vi "HFRR ADV v02.vi"() -> ()   [LabVIEW 2025] (continued)
        n1466 = local read "CAMERA ROI MIN TEMP"() -> (w1772:bool)
        n1467 = case shown="True" w1773 {
          selector: w1773 -> [_ w1780]
          frame False {
          }
          frame True {
            n1468 = Not(x=w1780) -> (.not. x?=w1779:bool)
            n1469 = local write "LIVE FEED MIN TEMP"(w1779) -> ()
            n1470 = call "CAMERA LIVE FEED FGV.vi"("Enum - Menu"=CAMERA_LIVE_FEED_ENUM."CAMERA MINIMIZE") -> ()  [unwired: 9 in, 2 out]
          }
        }
        n1471 = case shown="True" w1772 {
          selector: w1772 -> [_ w1777]
          frame False {
          }
          frame True {
            n1472 = Not(x=w1777) -> (.not. x?=w1776:bool)
            n1473 = local write "CAMERA ROI MIN TEMP"(w1776) -> ()
            n1474 = call "IMAGE ANALYSIS.vi"("Enum"=POST_ANALYSIS_ENUM."MINIMIZE UI") -> ()  [unwired: 9 in, 2 out]
          }
        }
        n1475 = local write "CAMERA ROI MAX TEMP"(TRUE ("CAMERA ROI MIN TEMP")) -> ()
      }
      frame "Advance" {
        n1476 = local read "LIVE FEED MIN TEMP"() -> (w1783:bool)
        n1477 = local write "LIVE FEED MAX TEMP"(TRUE ("LIVE FEED MAX TEMP")) -> ()
        n1478 = local read "CAMERA ROI MIN TEMP"() -> (w1781:bool)
        n1479 = case shown="True" w1783 {
          selector: w1783 -> [_ w1790]
          frame False {
          }
          frame True {
            n1480 = Not(x=w1790) -> (.not. x?=w1789:bool)
            n1481 = local write "LIVE FEED MIN TEMP"(w1789) -> ()
            n1482 = call "CAMERA LIVE FEED FGV.vi"("Enum - Menu"=CAMERA_LIVE_FEED_ENUM."CAMERA MINIMIZE") -> ()  [unwired: 9 in, 2 out]
          }
        }
        n1483 = local write "CAMERA ROI MAX TEMP"(TRUE ("CAMERA ROI MAX TEMP")) -> ()
        n1484 = case shown="True" w1781 {
          selector: w1781 -> [_ w1787]
          frame False {
          }
          frame True {
            n1485 = Not(x=w1787) -> (.not. x?=w1786:bool)
            n1486 = local write "CAMERA ROI MIN TEMP"(w1786) -> ()
            n1487 = call "IMAGE ANALYSIS.vi"("Enum"=POST_ANALYSIS_ENUM."MINIMIZE UI") -> ()  [unwired: 9 in, 2 out]
          }
        }
      }
      frame "Mooha" {
        n1488 = local read "LIVE FEED MIN TEMP"() -> (w1793:bool)
        n1489 = local write "LIVE FEED MAX TEMP"(TRUE ("LIVE FEED MAX TEMP")) -> ()
        n1490 = local read "CAMERA ROI MIN TEMP"() -> (w1791:bool)
        n1491 = case shown="True" w1793 {
          selector: w1793 -> [_ w1800]
          frame False {
          }
          frame True {
            n1492 = Not(x=w1800) -> (.not. x?=w1799:bool)
            n1493 = local write "LIVE FEED MIN TEMP"(w1799) -> ()
            n1494 = call "CAMERA LIVE FEED FGV.vi"("Enum - Menu"=CAMERA_LIVE_FEED_ENUM."CAMERA MINIMIZE") -> ()  [unwired: 9 in, 2 out]
          }
        }
        n1495 = local write "CAMERA ROI MAX TEMP"(TRUE ("CAMERA ROI MAX TEMP")) -> ()
        n1496 = case shown="True" w1791 {
          selector: w1791 -> [_ w1797]
          frame False {
          }
          frame True {
            n1497 = Not(x=w1797) -> (.not. x?=w1796:bool)
            n1498 = local write "CAMERA ROI MIN TEMP"(w1796) -> ()
            n1499 = call "IMAGE ANALYSIS.vi"("Enum"=POST_ANALYSIS_ENUM."MINIMIZE UI") -> ()  [unwired: 9 in, 2 out]
          }
        }
      }
    }
    n1500 = local read "Auto Start Test"() -> (w1537:bool)
    n1501 = case shown="True" "sign in temp" {
      frame False {
      }
      frame True {
        w1572 = 1 ("y")
        n1502 = local read "USERNAME"() -> (w1578:string)
        n1503 = local read "USER ID"() -> (w1575:string)
        n1504 = call <vilib>:"Trim Whitespace.vi"("string"=w1578) -> ("trimmed string"=w1577:string)  [unwired: 1 in]
        n1505 = call <vilib>:"Trim Whitespace.vi"("string"=w1575) -> ("trimmed string"=w1576:string)  [unwired: 1 in]
        n1506 = String Length(string=w1577) -> (length=w1574:i32)
        n1507 = String Length(string=w1576) -> (length=w1573:i32)
        n1508 = Greater?(x=w1574, y=w1572) -> (0:w1571:bool)
        n1509 = Greater?(x=w1573, y=w1572) -> (0:w1570:bool)
        n1510 = And(x=w1571, y=w1570) -> (x .and. y?=w1569:bool)
        n1511 = case shown="True" w1569 {
          frame False {
            n1512 = property on="Sign In" class="Bool (strict)"("DisabledEnum"=T19."Disabled" ("Disabled")) -> ()  [unwired: 2 in, 2 out]
          }
          frame True {
            n1513 = property on="Sign In" class="Bool (strict)"("DisabledEnum"=T19."Enabled" ("Disabled")) -> ()  [unwired: 2 in, 2 out]
          }
        }
      }
    }
    n1514 = local read "Air Temperature"() -> (w1554:bool)
    n1515 = local read "Coefficient Of Friction"() -> (w1555:bool)
    n1516 = case shown="False" w1537 {
      frame False {
        n1517 = local read "Auto stop temp"() -> (w1566:bool)
        n1518 = case shown="True" w1566 {
          frame False {
          }
          frame True {
            n1519 = local write "Auto Start Temp"(FALSE ("Auto Start Temp")) -> ()
          }
        }
      }
      frame True {
        "Auto stop temp" <- TRUE ("Auto stop temp")
      }
    }
    n1520 = local read "Humidity 3"() -> (w1553:bool)
    n1521 = case shown="\"HOME\"" w1563 {
      frame "HOME" {
        n1522 = local write "main tab sub"(enum32{"Page 1", "Page 2"}."Page 1" ("main tab sub")) -> ()
      }
      frame Default {
        n1523 = local write "main tab sub"(enum32{"Page 1", "Page 2"}."Page 2" ("main tab sub")) -> ()
      }
    }
    n1524 = case shown="True" w1562 {
      selector: w1562 -> [_ w1915]
      frame False {
      }
      frame True {
        n1525 = Not(x=w1915) -> (.not. x?=w1914:bool)
        n1526 = local write "Sign In"(w1914) -> ()
        n1527 = local write "Main Dashboard Buttons"(T25."Test Setup" ("Main Dashboard Buttons")) -> ()
      }
    }
    n1528 = case shown="\"Graph Display\"" "Num/Graph" {
      frame "Numeric Display", Default {
        n1529 = property on="Single/Multiple" class="RadioBtnsControl (strict)"("Visible"=FALSE) -> ()  [unwired: 2 in, 2 out]
        n1530 = property on="Single - Graph" class="Ring (strict)"("Visible"=FALSE) -> ()  [unwired: 2 in, 2 out]
        n1531 = local write "Main Tab Display"(T6."Dashboard 1" ("Main Tab Display")) -> ()
      }
      frame "Graph Display" {
        n1532 = property on="Single/Multiple" class="RadioBtnsControl (strict)"("Visible"=TRUE) -> ()  [unwired: 2 in, 2 out]
        n1533 = case shown="\"Multiple\"" "Single/Multiple" {
          frame "Single ", Default {
            n1534 = property on="Single - Graph" class="Ring (strict)"("Visible"=TRUE) -> ()  [unwired: 2 in, 2 out]
            n1535 = local write "Main Tab Display"(T6."Dashboard 3" ("Main Tab Display")) -> ()
          }
          frame "Multiple" {
            n1536 = property on="Single - Graph" class="Ring (strict)"("Visible"=FALSE) -> ()  [unwired: 2 in, 2 out]
            n1537 = local write "Main Tab Display"(T6."Dashboard 2" ("Main Tab Display")) -> ()
          }
        }
      }
    }
    n1538 = local read "Stroke"() -> (w1552:bool)
    n1539 = local read "USERNAME"() -> (w1557:string)
    n1540 = case shown="True" w1555 {
      selector: w1555 -> [_ w1840]
      frame False {
      }
      frame True {
        n1541 = Not(x=w1840) -> (.not. x?=w1839:bool)
        n1542 = local write "Coefficient Of Friction"(w1839) -> ()
        n1543 = local write "Tab Control 2"(T8."Coefficient Of Friction" ("Tab Control 2")) -> ()
      }
    }
    n1544 = case shown="True" w1554 {
      selector: w1554 -> [_ w1837]
      frame False {
      }
      frame True {
        n1545 = Not(x=w1837) -> (.not. x?=w1835:bool)
        n1546 = local write "Air Temperature"(w1835) -> ()
        n1547 = local write "Tab Control 2"(T8."Air Temperature" ("Tab Control 2")) -> ()
      }
    }
    n1548 = case shown="True" w1552 {
      selector: w1552 -> [_ w1831]
      frame False {
      }
      frame True {
        n1549 = Not(x=w1831) -> (.not. x?=w1829:bool)
        n1550 = local write "Stroke"(w1829) -> ()
        n1551 = local write "Tab Control 2"(T8."Stroke" ("Tab Control 2")) -> ()
      }
    }
    n1552 = local write "tested by"(w1557) -> ()
    n1553 = case shown="True" w1553 {
      selector: w1553 -> [_ w1834]
      frame False {
      }
      frame True {
        n1554 = Not(x=w1834) -> (.not. x?=w1832:bool)
        n1555 = local write "Humidity 3"(w1832) -> ()
        n1556 = local write "Tab Control 2"(T8."Humidity" ("Tab Control 2")) -> ()
      }
    }
    n1557 = case shown="\"Calibration\"" "Main Dashboard Buttons" {
      tunnel: [T4."HOME" ("Main Tab") T4."Test Setup" ("Main Tab") T4."Acquire" ("Main Tab") T4."Adv Scar" ("Main Tab") T4."Adv Scar Report" ("Main Tab") T4."Compare Files" ("Main Tab") T4."Calibration" ("Main Tab") T4."About" ("Main Tab") T4."Advance" ("Main Tab")] -> w1536
      frame "Home", Default {
      }
      frame "Test Setup" {
      }
      frame "Dashboard" {
      }
      frame "Imaging" {
      }
      frame "Report" {
      }
      frame "Analysis" {
      }
      frame "Calibration" {
      }
      frame "About" {
      }
      frame "Advance" {
      }
    }
    n1558 = Wait (ms)(milliseconds to wait=u32 100) -> ()  [unwired: 1 out]
    n1559 = local read "Main Tab Display"() -> (w1556:T6)
    n1560 = local write "Main Tab"(w1536) -> ()
    n1561 = case shown="\"Dashboard 3\"" w1556 {
      frame "Dashboard 1", Default {
        n1562 = property on="Reset Graph" class="Bool (strict)"("Visible"=FALSE) -> ()  [unwired: 2 in, 2 out]
      }
      frame "Dashboard 2" {
        n1563 = property on="Reset Graph" class="Bool (strict)"("Visible"=TRUE) -> ()  [unwired: 2 in, 2 out]
      }
      frame "Dashboard 3" {
        n1564 = property on="Reset Graph" class="Bool (strict)"("Visible"=TRUE) -> ()  [unwired: 2 in, 2 out]
      }
    }
    n1565 = local read "SCAR MEASURMENT"() -> (w1544:enum32{"Auto Scar", "Manual Scar"})
    n1566 = local read "Humidity"() -> (w1558:bool)
    n1567 = local read "Cap Live Image"() -> (w1541:bool)
    n1568 = local read "Sample Temperature"() -> (w1551:bool)
    n1569 = local read "Air Temp vs Humidity"() -> (w1549:bool)
    n1570 = local read "Frequency"() -> (w1550:bool)
    n1571 = case shown="False" w1558 {
      frame False {
        n1572 = local write "Humidity On Command"(TRUE ("Humidity On Command")) -> ()
        n1573 = case shown="True" "Humidity Off Command" {
          selector: "Humidity Off Command" -> [_ w1847]
          frame False {
          }
          frame True {
            n1574 = stacked-sequence {
              frame #0 {
                n1575 = local read "WriteHumidity"() -> (w1849:string[])
                n1576 = Insert Into Array(array=w1849, new element="R;1" ("new element/subarray")) -> (w1848:string[])  [unwired: 1 in]
                n1577 = local write "WriteHumidity"(w1848) -> ()
              }
              frame #1 {
                n1578 = Wait (ms)(milliseconds to wait=u32 500) -> ()  [unwired: 1 out]
              }
              frame #2 {
                n1579 = local read "WriteHumidity"() -> (w1853:string[])
                n1580 = local read "EVENT LOG"() -> (w1857:string)
                n1581 = call "Event Log.vi"("Content"="Humidity Control Off" ("string"), "EVENT LOG"=w1857) -> ("EVENT LOG"=w1858:string)  [unwired: 8 in, 1 out]
                n1582 = local write "EVENT LOG"(w1858) -> ()
                n1583 = Insert Into Array(array=w1853, new element="R;1" ("new element/subarray")) -> (w1854:string[])  [unwired: 1 in]
                n1584 = local write "WriteHumidity"(w1854) -> ()
                n1585 = local write "Humidity 2"(TRUE ("Humidity")) -> ()
              }
            }
            n1586 = Not(x=w1847) -> (.not. x?=w1846:bool)
            n1587 = local write "Humidity Off Command"(w1846) -> ()
          }
        }
      }
      frame True {
        n1588 = local write "Humidity Off Command"(TRUE ("Humidity Off Command")) -> ()
        n1589 = case shown="False" "Humidity On Command" {
          selector: "Humidity On Command" -> [_ w1862]
          frame False {
          }
          frame True {
            n1590 = stacked-sequence {
              frame #0 {
                n1591 = local read "Set Rh"() -> (w1868:dbl)
                n1592 = local read "WriteHumidity"() -> (w1864:string[])
                n1593 = Number To Fractional String(number=w1868, precision (6)=i16 2) -> (F-format string=w1869:string)  [unwired: 2 in]
                n1594 = Concatenate Strings("M;" ("new element/subarray"), w1869) -> (w1867:string)
                n1595 = Insert Into Array(array=w1864, new element=w1867) -> (w1863:string[])  [unwired: 1 in]
                n1596 = local write "WriteHumidity"(w1863) -> ()
              }
              frame #1 {
                n1597 = Wait (ms)(milliseconds to wait=u32 500) -> ()  [unwired: 1 out]
              }
              frame #2 {
                n1598 = local read "WriteHumidity"() -> (w1872:string[])
                n1599 = local read "Set Rh"() -> (w1876:dbl)
                n1600 = Number To Fractional String(number=w1876, precision (6)=i16 2) -> (F-format string=w1877:string)  [unwired: 2 in]
                n1601 = Concatenate Strings("M;" ("new element/subarray"), w1877) -> (w1875:string)
                n1602 = Insert Into Array(array=w1872, new element=w1875) -> (w1871:string[])  [unwired: 1 in]
                n1603 = local write "WriteHumidity"(w1871) -> ()
              }
              frame #3 {
                n1604 = Wait (ms)(milliseconds to wait=u32 500) -> ()  [unwired: 1 out]
              }
              frame #4 {
                (unwired) "% RH" ("string")
                (unwired) i16 2 ("precision (6)")
                (unwired) "M;" ("new element/subarray")
                n1605 = local read "Set Rh"() -> (w1886:dbl)
                n1606 = local read "WriteHumidity"() -> (w1879:string[])
                n1607 = Number To Fractional String(number=w1886, precision (6)=i16 2) -> (F-format string=w1883:string)  [unwired: 2 in]
                n1608 = Concatenate Strings("M;" ("new element/subarray"), w1883) -> (w1887:string)
                n1609 = Concatenate Strings("Humidity Set to : " ("string"), w1883, "% RH" ("string")) -> (w1881:string)
                n1610 = Insert Into Array(array=w1879, new element=w1887) -> (w1880:string[])  [unwired: 1 in]
                n1611 = disable-structure shown="Enabled" {
                  frame Enabled {
                    n1612 = local read "EVENT LOG"() -> (w1890:string)
                    n1613 = call "Event Log.vi"("Content"="Humidity Control On", "EVENT LOG"=w1890) -> ("EVENT LOG"=w1891:string)  [unwired: 8 in, 1 out]
                    n1614 = local write "EVENT LOG"(w1891) -> ()
                  }
                  frame Disabled {
                  }
                }
                n1615 = disable-structure shown="Enabled" {
                  disable-tunnel: w1881 -> [_ _]
                  frame Enabled {
                    n1616 = local read "EVENT LOG"() -> (w1893:string)
                    n1617 = call "Event Log.vi"("Content"="Humidity Control On", "EVENT LOG"=w1893) -> ("EVENT LOG"=w1894:string)  [unwired: 8 in, 1 out]
                    n1618 = local write "EVENT LOG"(w1894) -> ()
                  }
                  frame Disabled {
                  }
                }
                n1619 = local write "WriteHumidity"(w1880) -> ()
              }
            }
            n1620 = Not(x=w1862) -> (.not. x?=w1861:bool)
            n1621 = local write "Humidity On Command"(w1861) -> ()
          }
        }
      }
    }
    n1622 = Equal?(x=w1544, y=enum32{"Auto Scar", "Manual Scar"}."Auto Scar" ("SCAR MEASURMENT")) -> (x = y?=w1540:bool)
    n1623 = local read "TEST STANDARD"() -> (w1547:T5)
    n1624 = And(x=w1541, y=w1540) -> (x .and. y?=w1542:bool)
    n1625 = case shown="True" w1542 {
      selector: w1542 -> [_ w1645]
      tunnel: errorcluster {"status"=FALSE, "code"=0, "source"=""} ("error in (no error) 3") -> [_ w1646]
      frame False {
      }
      frame True {
        n1626 = stacked-sequence {
          tunnel: w1646 -> [_ _ _ _ _ _ _ w1695]
          tunnel: w1645 -> [_ _ _ _ _ w1675 _ _]
          frame #0 {
            n1627 = call "CAMERA LIVE FEED FGV.vi"("Enum - Menu"=CAMERA_LIVE_FEED_ENUM."CAMERA MINIMIZE") -> ()  [unwired: 9 in, 2 out]
          }
          frame #1 {
            n1628 = property on="Auto Scar Check  2" class="Clust (strict)"("Visible"=TRUE) -> ()  [unwired: 2 in, 2 out]
          }
          frame #2 {
            n1629 = String To Path(string="C:\\LAB-IQ\\Image Calibrate v01.dcf") -> (path=w1651:path)
            n1630 = Open/Create/Replace File ("Open File")(file path (use dialog)=w1651) -> (refnum out=w1652:refnum<file>)  [unwired: 5 in, 2 out]
            n1631 = for {
              N: 4 -> [_]
              tunnel: w1652 -> [w1658]
              i -> [w1654]
              n1632 = Read from Text File ("Read File")(file (use dialog)=w1658) -> (text=w1659:string)  [unwired: 3 in, 3 out]
              n1633 = String Subset(string=w1659, offset (0)=6, length (rest)=10 ("length (rest)")) -> (substring=w1655:string)
              n1634 = Fract/Exp String To Number(string=w1655) -> (number=w1653:dbl)  [unwired: 3 in, 1 out]
              n1635 = case shown="0" w1654 {
                tunnel: w1653 -> [w1660 w1661 _ w1662 _]
                frame 0 {
                  "5x Gain" <- w1660
                }
                frame 1 {
                  "10x Gain" <- w1661
                }
                frame 2 {
                }
                frame 3 {
                  "100x gain" <- w1662
                }
                frame 4, Default {
                }
              }
            }
          }
          frame #3 {
            n1636 = local read "FILE 3"() -> (w1668:string)
            n1637 = call <vilib>:"Trim Whitespace.vi"("string"="C:\\LAB-IQ\\images\\") -> ("trimmed string"=w1670:string)  [unwired: 1 in]
            n1638 = String To Path(string=w1670) -> (path=w1669:path)
            n1639 = Concatenate Strings(w1668, ".png" ("string")) -> (w1667:string)
            n1640 = Build Path(base path=w1669, name or relative path=w1667) -> (appended path=w1665:path)
            "Image path" <- w1665
            n1641 = Path To String(path=w1665) -> (string=w1664:string)
            n1642 = call "CAMERA LIVE FEED FGV.vi"("Enum - Menu"=CAMERA_LIVE_FEED_ENUM."CAMERA SAVE", "Image Path"=w1664) -> ()  [unwired: 8 in, 2 out]
          }
          frame #4 {
            n1643 = One Button Dialog(message="Image saved successfully") -> ()  [unwired: 1 in, 1 out]
          }
          frame #5 {
            n1644 = local read "TEST STANDARD"() -> (w1674:T5)
            n1645 = local read "Magnification len live scar"() -> (w1686:string)
            n1646 = Not(x=w1675) -> (.not. x?=w1676:bool)
            n1647 = local write "Cap Live Image"(w1676) -> ()
            n1648 = case shown="\"ASTM D7688\"" w1674 {
              tunnel: ["ASTM D6079" "ISO 12156" "ASTM D7688"] -> w1673
              frame "ASTM D6079", Default {
              }
              frame "ISO 12156" {
              }
              frame "ASTM D7688" {
              }
            }
            n1649 = case shown="\"5x\", Default" w1686 {
              tunnel: [w1690 w1691] -> w1685
              frame "5x", Default {
                n1650 = local read "5x Gain"() -> (w1690:dbl)
              }
              frame "10x" {
                # "5x"
                n1651 = local read "10x Gain"() -> (w1691:dbl)
              }
            }
            n1652 = local read "Image path"() -> (w1684:path)
            n1653 = local read "FILE 3"() -> (w1677:string)
            n1654 = call "EDGE DETCTION.vi"("GAIN VALUE"=w1685, "Image Path"=w1684) -> ("error out"=w1683:errorcluster, "return value"=w1682:cluster{string, string, dbl, dbl, dbl})  [unwired: 8 in]
            n1655 = Bundle By Name(cluster=T26 {"File Name"="", "Test Method"="", "Operator"="", "Fuel Description"="", "Date and time"=""} ("Main Ref"), "File Name"=w1677, "Test Method"=w1673) -> (w1678:T26)
            n1656 = call "duf file read.vi"("error in (no error)"=w1683, "Main Ref"=w1678) -> ("error out"=w1681:errorcluster, "Main Ref 2"=w1679:T26)  [unwired: 7 in, 1 out]
            n1657 = call "EDGE DETECTION REPORT.vi"("error in (no error)"=w1681, "return value 2"=w1682, "Main Ref"=w1679) -> ()  [unwired: 8 in, 1 out]
          }
          frame #6 {
            n1658 = property on="Auto Scar Check  2" class="Clust (strict)"("Visible"=FALSE) -> ()  [unwired: 2 in, 2 out]
          }
          frame #7 {
            n1659 = call "CAMERA LIVE FEED FGV.vi"("Enum - Menu"=CAMERA_LIVE_FEED_ENUM."CAMERA MINIMIZE", "error in (no error)"=w1695) -> ()  [unwired: 8 in, 2 out]
            n1660 = local write "Main Dashboard Buttons"(T1."Home" ("Main Dashboard Buttons")) -> ()
            n1661 = local write "Main Tab"(T4."HOME" ("Main Tab")) -> ()
          }
        }
      }
    }
    n1662 = local read "Heater Button"() -> (w1548:bool)
    n1663 = case shown="True" w1550 {
      selector: w1550 -> [_ w1825]
      frame False {
      }
      frame True {
        n1664 = Not(x=w1825) -> (.not. x?=w1823:bool)
        n1665 = local write "Frequency"(w1823) -> ()
        n1666 = local write "Tab Control 2"(T8."Frequency" ("Tab Control 2")) -> ()
      }
    }
    n1667 = case shown="True" w1549 {
      selector: w1549 -> [_ w1822]
      frame False {
      }
      frame True {
        n1668 = Not(x=w1822) -> (.not. x?=w1820:bool)
        n1669 = local write "Air Temp vs Humidity"(w1820) -> ()
        n1670 = local write "Tab Control 2"(T8."Air Temp vs Rh" ("Tab Control 2")) -> ()
      }
    }
    n1671 = case shown="True" w1551 {
      selector: w1551 -> [_ w1828]
      frame False {
      }
      frame True {
        n1672 = Not(x=w1828) -> (.not. x?=w1826:bool)
        n1673 = local write "Sample Temperature"(w1826) -> ()
        n1674 = local write "Tab Control 2"(T8."Sample Temperature" ("Tab Control 2")) -> ()
      }
    }
    n1675 = case shown="\"ASTM D7688\"" w1547 {
      frame "ASTM D6079", Default {
        w1801 = "ASTM D6079 TEST CONDITIONS" ("Standard 2")
        n1676 = local write "Standard 2"(w1801) -> ()
        n1677 = local write "Standard"(w1801) -> ()
      }
      frame "ISO 12156" {
        w1802 = "ISO 12156 TEST CONDITIONS" ("Standard 2")
        n1678 = local write "Standard 2"(w1802) -> ()
        n1679 = local write "Standard"(w1802) -> ()
      }
      frame "ASTM D7688" {
        w1803 = "ASTM D7688 TEST CONDITIONS" ("Standard 2")
        n1680 = local write "Standard 2"(w1803) -> ()
        n1681 = local write "Standard"(w1803) -> ()
      }
      frame "Custom" {
        w1804 = "CUSTOM TEST CONDITIONS" ("Standard 2")
        n1682 = local write "Standard 2"(w1804) -> ()
        n1683 = local write "Standard"(w1804) -> ()
      }
    }
    n1684 = case shown="True" w1548 {
      frame False {
        n1685 = local write "Temperature On Command"(TRUE ("Temperature On Command")) -> ()
        n1686 = case shown="True" "Temperature Off Command" {
          selector: "Temperature Off Command" -> [_ w1808]
          frame False {
          }
          frame True {
            n1687 = Not(x=w1808) -> (.not. x?=w1807:bool)
            n1688 = local read "EVENT LOG"() -> (w1811:string)
            n1689 = local write "Temperature Off Command"(w1807) -> ()
            n1690 = call "Event Log.vi"("Content"="Heater Off", "EVENT LOG"=w1811) -> ("EVENT LOG"=w1810:string)  [unwired: 8 in, 1 out]
            n1691 = local write "EVENT LOG"(w1810) -> ()
          }
        }
      }
      frame True {
        n1692 = local write "Temperature Off Command"(TRUE ("Temperature Off Command")) -> ()
        n1693 = case shown="True" "Temperature On Command" {
          selector: "Temperature On Command" -> [_ w1815]
          frame False {
          }
          frame True {
            n1694 = Not(x=w1815) -> (.not. x?=w1814:bool)
            n1695 = local write "Temperature On Command"(w1814) -> ()
            n1696 = disable-structure shown="Enabled" {
              disable-tunnel: "Heater On" -> [w1817 _]
              frame Enabled {
                n1697 = local read "EVENT LOG"() -> (w1818:string)
                n1698 = call "Event Log.vi"("Content"=w1817, "EVENT LOG"=w1818) -> ("EVENT LOG"=w1819:string)  [unwired: 8 in, 1 out]
                n1699 = local write "EVENT LOG"(w1819) -> ()
              }
              frame Disabled {
              }
            }
          }
        }
      }
    }
    n1700 = local read "Main Tab"() -> (w1539:T4)
    n1701 = case shown="\"About\"" w1539 {
      frame "HOME", Default {
        w1581 = T19."Enabled" ("Disabled")
        n1702 = local read "Service Password enable"() -> (w1583:bool)
        n1703 = property on="Imaging" class="Bool (strict)"("DisabledEnum"=w1581) -> ()  [unwired: 2 in, 2 out]
        n1704 = property on="Dashboard" class="Bool (strict)"("DisabledEnum"=w1581) -> ()  [unwired: 2 in, 2 out]
        n1705 = property on="Test Setup" class="Bool (strict)"("DisabledEnum"=w1581) -> ()  [unwired: 2 in, 2 out]
        n1706 = property on="Analysis" class="Bool (strict)"("DisabledEnum"=w1581) -> ()  [unwired: 2 in, 2 out]
        n1707 = property on="Home" class="Bool (strict)"("DisabledEnum"=w1581) -> ()  [unwired: 2 in, 2 out]
        n1708 = property on="Report" class="Bool (strict)"("DisabledEnum"=w1581) -> ()  [unwired: 2 in, 2 out]
        n1709 = property on="Main Dashboard Buttons" class="RadioBtnsControl (strict)"("DisabledEnum"=w1581) -> ()  [unwired: 2 in, 2 out]
        n1710 = property on="Calibration" class="Bool (strict)"("DisabledEnum"=w1581) -> ()  [unwired: 2 in, 2 out]
        n1711 = case shown="True" w1583 {
          tunnel: [T19."Disabled" ("Disabled") T19."Enabled" ("Disabled")] -> w1582
          frame False {
          }
          frame True {
          }
        }
        n1712 = property on="About" class="Bool (strict)"("DisabledEnum"=w1582) -> ()  [unwired: 2 in, 2 out]
      }
      frame "Test Setup" {
        w1588 = T19."Enabled" ("Disabled")
        n1713 = local read "Service Password enable"() -> (w1587:bool)
        n1714 = property on="Dashboard" class="Bool (strict)"("DisabledEnum"=T19."Disabled" ("Disabled")) -> ()  [unwired: 2 in, 2 out]
        n1715 = property on="Imaging" class="Bool (strict)"("DisabledEnum"=w1588) -> ()  [unwired: 2 in, 2 out]
        n1716 = property on="Analysis" class="Bool (strict)"("DisabledEnum"=w1588) -> ()  [unwired: 2 in, 2 out]
        n1717 = property on="Home" class="Bool (strict)"("DisabledEnum"=w1588) -> ()  [unwired: 2 in, 2 out]
        n1718 = property on="Report" class="Bool (strict)"("DisabledEnum"=w1588) -> ()  [unwired: 2 in, 2 out]
        n1719 = property on="Test Setup" class="Bool (strict)"("DisabledEnum"=w1588) -> ()  [unwired: 2 in, 2 out]
        n1720 = case shown="True" w1587 {
          tunnel: [T19."Disabled" ("Disabled") T19."Enabled" ("Disabled")] -> w1586
          frame False {
          }
          frame True {
          }
        }
        n1721 = property on="About" class="Bool (strict)"("DisabledEnum"=w1586) -> ()  [unwired: 2 in, 2 out]
      }
      frame "Adv Scar" {
        w1595 = T19."Enabled" ("Disabled")
        n1722 = property on="Dashboard" class="Bool (strict)"("DisabledEnum"=T19."Disabled" ("Disabled")) -> ()  [unwired: 2 in, 2 out]
        n1723 = property on="Imaging" class="Bool (strict)"("DisabledEnum"=w1595) -> ()  [unwired: 2 in, 2 out]
        n1724 = property on="Analysis" class="Bool (strict)"("DisabledEnum"=w1595) -> ()  [unwired: 2 in, 2 out]
        n1725 = property on="Home" class="Bool (strict)"("DisabledEnum"=w1595) -> ()  [unwired: 2 in, 2 out]
        n1726 = property on="Report" class="Bool (strict)"("DisabledEnum"=w1595) -> ()  [unwired: 2 in, 2 out]
        n1727 = property on="Test Setup" class="Bool (strict)"("DisabledEnum"=w1595) -> ()  [unwired: 2 in, 2 out]
        n1728 = local read "Service Password enable"() -> (w1593:bool)
        n1729 = case shown="True" w1593 {
          tunnel: [T19."Disabled" ("Disabled") T19."Enabled" ("Disabled")] -> w1592
          frame False {
          }
          frame True {
          }
        }
        n1730 = property on="About" class="Bool (strict)"("DisabledEnum"=w1592) -> ()  [unwired: 2 in, 2 out]
      }
      frame "Calibration" {
        w1598 = T19."Enabled" ("Disabled")
        n1731 = property on="Dashboard" class="Bool (strict)"("DisabledEnum"=T19."Disabled" ("Disabled")) -> ()  [unwired: 2 in, 2 out]
        n1732 = property on="Imaging" class="Bool (strict)"("DisabledEnum"=w1598) -> ()  [unwired: 2 in, 2 out]
        n1733 = property on="Analysis" class="Bool (strict)"("DisabledEnum"=w1598) -> ()  [unwired: 2 in, 2 out]
        n1734 = property on="Home" class="Bool (strict)"("DisabledEnum"=w1598) -> ()  [unwired: 2 in, 2 out]
        n1735 = property on="Report" class="Bool (strict)"("DisabledEnum"=w1598) -> ()  [unwired: 2 in, 2 out]
        n1736 = property on="Test Setup" class="Bool (strict)"("DisabledEnum"=w1598) -> ()  [unwired: 2 in, 2 out]
        n1737 = local read "Service Password enable"() -> (w1600:bool)
        n1738 = property on="Calibration" class="Bool (strict)"("DisabledEnum"=w1598) -> ()  [unwired: 2 in, 2 out]
        n1739 = case shown="True" w1600 {
          tunnel: [T19."Disabled" ("Disabled") T19."Enabled" ("Disabled")] -> w1599
          frame False {
          }
          frame True {
          }
        }
        n1740 = property on="About" class="Bool (strict)"("DisabledEnum"=w1599) -> ()  [unwired: 2 in, 2 out]
      }
      frame "Adv Scar Report" {
        w1606 = T19."Enabled" ("Disabled")
        n1741 = property on="Dashboard" class="Bool (strict)"("DisabledEnum"=T19."Disabled" ("Disabled")) -> ()  [unwired: 2 in, 2 out]
        n1742 = property on="Imaging" class="Bool (strict)"("DisabledEnum"=w1606) -> ()  [unwired: 2 in, 2 out]
        n1743 = property on="Analysis" class="Bool (strict)"("DisabledEnum"=w1606) -> ()  [unwired: 2 in, 2 out]
        n1744 = property on="Home" class="Bool (strict)"("DisabledEnum"=w1606) -> ()  [unwired: 2 in, 2 out]
        n1745 = property on="Report" class="Bool (strict)"("DisabledEnum"=w1606) -> ()  [unwired: 2 in, 2 out]
        n1746 = property on="Test Setup" class="Bool (strict)"("DisabledEnum"=w1606) -> ()  [unwired: 2 in, 2 out]
        n1747 = local read "Service Password enable"() -> (w1605:bool)
        n1748 = case shown="True" w1605 {
          tunnel: [T19."Disabled" ("Disabled") T19."Enabled" ("Disabled")] -> w1604
          frame False {
          }
          frame True {
          }
        }
        n1749 = property on="About" class="Bool (strict)"("DisabledEnum"=w1604) -> ()  [unwired: 2 in, 2 out]
      }
      frame "Compare Files" {
        w1612 = T19."Enabled" ("Disabled")
        n1750 = local read "Service Password enable"() -> (w1611:bool)
        n1751 = property on="Dashboard" class="Bool (strict)"("DisabledEnum"=T19."Disabled" ("Disabled")) -> ()  [unwired: 2 in, 2 out]
        n1752 = property on="Imaging" class="Bool (strict)"("DisabledEnum"=w1612) -> ()  [unwired: 2 in, 2 out]
        n1753 = property on="Analysis" class="Bool (strict)"("DisabledEnum"=w1612) -> ()  [unwired: 2 in, 2 out]
        n1754 = property on="Home" class="Bool (strict)"("DisabledEnum"=w1612) -> ()  [unwired: 2 in, 2 out]
        n1755 = property on="Report" class="Bool (strict)"("DisabledEnum"=w1612) -> ()  [unwired: 2 in, 2 out]
        n1756 = property on="Test Setup" class="Bool (strict)"("DisabledEnum"=w1612) -> ()  [unwired: 2 in, 2 out]
        n1757 = case shown="True" w1611 {
          tunnel: [T19."Disabled" ("Disabled") T19."Enabled" ("Disabled")] -> w1610
          frame False {
          }
          frame True {
          }
        }
        n1758 = property on="About" class="Bool (strict)"("DisabledEnum"=w1610) -> ()  [unwired: 2 in, 2 out]
      }
      frame "Acquire" {
        n1759 = local read "Service Password enable"() -> (w1617:bool)
        n1760 = property on="Test Setup" class="Bool (strict)"("DisabledEnum"=T19."Disabled" ("Disabled")) -> ()  [unwired: 2 in, 2 out]
        n1761 = local read "Auto Start Test"() -> (w1619:bool)
        n1762 = local read "RUN"() -> (w1621:bool)
        n1763 = case shown="True" w1617 {
          tunnel: [T19."Disabled" ("Disabled") T19."Enabled" ("Disabled")] -> w1618
          frame False {
          }
          frame True {
          }
        }
        n1764 = Or(x=w1621, y=w1619) -> (x .or. y?=w1620:bool)
        n1765 = case shown="True" w1620 {
          tunnel: [T19."Enabled" ("Disabled") T19."Disabled" ("Disabled")] -> w1616
          frame False {
          }
          frame True {
          }
        }
        n1766 = property on="About" class="Bool (strict)"("DisabledEnum"=w1618) -> ()  [unwired: 2 in, 2 out]
        n1767 = property on="Imaging" class="Bool (strict)"("DisabledEnum"=w1616) -> ()  [unwired: 2 in, 2 out]
        n1768 = property on="Dashboard" class="Bool (strict)"("DisabledEnum"=w1616) -> ()  [unwired: 2 in, 2 out]
        n1769 = property on="Analysis" class="Bool (strict)"("DisabledEnum"=w1616) -> ()  [unwired: 2 in, 2 out]
        n1770 = property on="Home" class="Bool (strict)"("DisabledEnum"=w1616) -> ()  [unwired: 2 in, 2 out]
        n1771 = property on="Report" class="Bool (strict)"("DisabledEnum"=w1616) -> ()  [unwired: 2 in, 2 out]
        n1772 = property on="Calibration" class="Bool (strict)"("DisabledEnum"=w1616) -> ()  [unwired: 2 in, 2 out]
      }
      frame "About" {
        n1773 = local read "FILE"() -> (w1635:string)
        n1774 = local read "TEST FILE NAM,E SAVED"() -> (w1628:bool)
        n1775 = call <vilib>:"Trim Whitespace.vi"("string"=w1635) -> ("trimmed string"=w1634:string)  [unwired: 1 in]
        n1776 = local read "Auto Start Test"() -> (w1638:bool)
        n1777 = String Length(string=w1634) -> (length=w1633:i32)
        n1778 = Greater?(x=w1633, y=1) -> (0:w1630:bool)
        n1779 = And(x=w1630, y=w1628) -> (x .and. y?=w1629:bool)
        n1780 = local read "RUN"() -> (w1640:bool)
        n1781 = case shown="True" w1629 {
          tunnel: [T19."Disabled" ("Disabled") T19."Enabled" ("Disabled")] -> w1631
          frame False {
          }
          frame True {
          }
        }
        n1782 = Or(x=w1640, y=w1638) -> (x .or. y?=w1639:bool)
        n1783 = property on="About" class="Bool (strict)"("DisabledEnum"=T19."Enabled" ("Disabled")) -> ()  [unwired: 2 in, 2 out]
        n1784 = case shown="False" w1639 {
          tunnel: [T19."Enabled" ("Disabled") T19."Disabled" ("Disabled")] -> w1637
          frame False {
          }
          frame True {
          }
        }
        n1785 = property on="Dashboard" class="Bool (strict)"("DisabledEnum"=w1631) -> ()  [unwired: 2 in, 2 out]
        n1786 = property on="Test Setup" class="Bool (strict)"("DisabledEnum"=T19."Disabled" ("Disabled")) -> ()  [unwired: 2 in, 2 out]
        n1787 = property on="Imaging" class="Bool (strict)"("DisabledEnum"=w1637) -> ()  [unwired: 2 in, 2 out]
        n1788 = property on="Analysis" class="Bool (strict)"("DisabledEnum"=w1637) -> ()  [unwired: 2 in, 2 out]
        n1789 = property on="Home" class="Bool (strict)"("DisabledEnum"=w1637) -> ()  [unwired: 2 in, 2 out]
        n1790 = property on="Report" class="Bool (strict)"("DisabledEnum"=w1637) -> ()  [unwired: 2 in, 2 out]
      }
    }
    n1791 = local read "Quit"() -> (w1565:bool)
    "Single" <- "Single - Graph"
  }
  n1792 = disable-structure shown="Disabled" {
    disable-tunnel: [w1919 _] -> w47
    disable-tunnel: _ -> [w1918 _]
    frame Disabled {
      n1793 = while {
        tunnel: w1918 -> [_]
        tunnel: [w1920] -> w1919
        tunnel: [w1921] -> _
        i -> [w1921]
        stop <- w1920 stop-if-true
        w1937 = u16 10 items=["1.0"=10, "1.5"=15, "2.0"=20] ("stop bits (10: 1 bit)")
        n1794 = Wait (ms)(milliseconds to wait=u32 10) -> ()  [unwired: 1 out]
        n1795 = call-poly "VISA Configure Serial Port"("VISA resource name"=refnum<visa-resource-name> "ASRL1::INSTR" ("COM PORT"), "timeout (10sec)"=u32 10, "baud rate (9600)"=u32 57600, "data bits (8)"=u16 8, "stop bits (10: 1 bit)"=w1937) -> ("VISA resource name out"=w1923:refnum<visa-resource-name>, "error out"=w1932:errorcluster)  [unwired: 9 in]
        n1796 = VISA Read(VISA resource name=w1923, byte count=u32 2 ("byte count (0)")) -> (read buffer=w1931:string)  [unwired: 1 in, 3 out]
        n1797 = String Subset(string=w1931, offset (0)=0, length (rest)=2 ("length (rest)")) -> (substring=w1930:string)
        n1798 = Match Pattern(string=w1930, regular expression="<>") -> (offset past match=w1927:i32)  [unwired: 1 in, 3 out]
        n1799 = Greater Or Equal?(x=w1927, y=0) -> (x >= y?=w1922:bool)
        n1800 = case shown="True" w1922 {
          tunnel: w1923 -> [_ w1941]
          tunnel: w1932 -> [_ w1940]
          frame False {
          }
          frame True {
            n1801 = VISA Read(VISA resource name=w1941, byte count=u32 32 ("byte count (0)"), error in (no error)=w1940) -> (read buffer=w1939:string)  [unwired: 3 out]
            n1802 = String Subset(string=w1939, offset (0)=0, length (rest)=8 ("length (rest)")) -> (substring=w1943:string)
            n1803 = String Subset(string=w1939, offset (0)=8, length (rest)=8 ("length (rest)")) -> (substring=w1944:string)
            n1804 = Decimal String To Number(string=w1944) -> (number=w1951:i32)  [unwired: 2 in, 1 out]
            n1805 = Decimal String To Number(string=w1943) -> (number=w1947:i32)  [unwired: 2 in, 1 out]
            n1806 = Divide(x=w1951, y=10000) -> ()  [unwired: 1 out]
            n1807 = Divide(x=w1947, y=1000000) -> ()  [unwired: 1 out]
          }
        }
        n1808 = local read "Quit"() -> (w1920:bool)
      }
    }
    frame Enabled {
    }
  }
  n1809 = Tick Count (ms)() -> (millisecond timer value=w9:u32)
  n1810 = while {
    shift-right: [w1999] -> _
    shift-left: w11 -> [w2003]
    shift-right: [w1998] -> _
    shift-left: w10 -> [w2002]
    shift-right: [w1997] -> _
    shift-left: w11 -> [w2001]
    shift-right: [w1996] -> _
    shift-left: w10 -> [w2000]
    shift-right: [w1994] -> _
    shift-left: w9 -> [w1995]
    shift-right: [w1991] -> _
    shift-left: w1 -> [w1992]
    shift-right: [w1990] -> _
    shift-left: w1 -> [w1993]
    shift-right: [w1983] -> _
    shift-left: w1 -> [w1989]
    shift-right: [w1982] -> _
    shift-left: w1 -> [w1988]
    shift-right: [w1981] -> _
    shift-left: w1 -> [w1987]
    shift-right: [w1980] -> _
    shift-left: w1 -> [w1986]
    shift-right: [w1979] -> _
    shift-left: w1 -> [w1985]
    shift-right: [w1978] -> _
    shift-left: w1 -> [w1984]
    shift-right: [w1977] -> _
    shift-left: w1 -> [w1971]
    shift-right: [w1976] -> _
    shift-left: w1 -> [w1970]
    shift-right: [w1975] -> _
    shift-left: w1 -> [w1969]
    shift-right: [w1974] -> _
    shift-left: w1 -> [w1968]
    shift-right: [w1973] -> _
    shift-left: w1 -> [w1967]
    shift-right: [w1972] -> _
    shift-left: w1 -> [w1966]
    shift-right: [w1958] -> _
    shift-left: w1 -> [w1961]
    shift-right: [w1957] -> _
    shift-left: w1 -> [w1960]
    shift-right: [w1956] -> _
    shift-left: w1 -> [w1959]
    shift-right: [w1953] -> _
    shift-left: w1 -> [w1954]
    stop <- w2005 stop-if-true
    n1811 = local read "Read UNO"() -> (w1965:string)
    n1812 = local read "Error  2"() -> (w2004:errorcluster)
    n1813 = call <vilib>:"Trim Whitespace.vi"("string"=w1965) -> ("trimmed string"=w1955:string)  [unwired: 1 in]
    n1814 = String Length(string=w1955) -> (length=w1964:i32)
    n1815 = Greater Or Equal?(x=w1964, y=17) -> (x >= y?=w1962:bool)
    n1816 = case shown="No Error" w2004 {
      tunnel: w2003 -> [w2053 w2153]
      tunnel: w2002 -> [w2052 w2152]
      tunnel: w2001 -> [w2051 w2151]
      tunnel: w2000 -> [w2050 w2150]
      tunnel: [w2049 w2153] -> w1999
      tunnel: [w2048 w2152] -> w1998
      tunnel: [w2047 w2151] -> w1997
      tunnel: [w2046 w2150] -> w1996
      tunnel: w1995 -> [w2045 w2149]
      tunnel: [w2044 w2149] -> w1994
      tunnel: w1992 -> [w2043 w2148]
      tunnel: w1993 -> [w2042 w2147]
      tunnel: [w2041 w2148] -> w1991
      tunnel: [w2040 w2147] -> w1990
      tunnel: w1989 -> [w2039 w2146]
      tunnel: w1988 -> [w2038 w2145]
      tunnel: w1987 -> [w2037 w2144]
      tunnel: w1986 -> [w2036 w2143]
      tunnel: w1985 -> [w2035 w2142]
      tunnel: w1984 -> [w2034 w2141]
      tunnel: [w2033 w2146] -> w1983
      tunnel: [w2032 w2145] -> w1982
      tunnel: [w2031 w2144] -> w1981
      tunnel: [w2030 w2143] -> w1980
      tunnel: [w2029 w2142] -> w1979
      tunnel: [w2028 w2141] -> w1978
      tunnel: w1971 -> [w2027 w2140]
      tunnel: [w2026 w2140] -> w1977
      tunnel: [w2025 w2136] -> w1976
      tunnel: [w2024 w2135] -> w1975
      tunnel: [w2023 w2139] -> w1974
      tunnel: [w2022 w2138] -> w1973
      tunnel: [w2021 w2137] -> w1972
      tunnel: w1970 -> [w2020 w2139]
      tunnel: w1969 -> [w2019 w2138]
      tunnel: w1968 -> [w2018 w2137]
      tunnel: w1967 -> [w2017 w2136]
      tunnel: w1966 -> [w2016 w2135]
      tunnel: w1955 -> [w2015 _]
      tunnel: w1962 -> [w2014 _]
      tunnel: w1961 -> [w2013 w2134]
      tunnel: w1960 -> [w2012 w2133]
      tunnel: w1959 -> [w2011 w2132]
      tunnel: [w2010 w2134] -> w1958
      tunnel: [w2009 w2133] -> w1957
      tunnel: [w2008 w2132] -> w1956
      tunnel: w1954 -> [w2007 w2131]
      tunnel: [w2006 w2131] -> w1953
      frame No Error {
        n1817 = case shown="True" w2014 {
          tunnel: w2053 -> [w2070 w2124]
          tunnel: w2052 -> [w2069 w2123]
          tunnel: w2051 -> [w2068 w2122]
          tunnel: w2050 -> [w2067 w2121]
          tunnel: [w2070 w2120] -> w2049
          tunnel: [w2069 w2119] -> w2048
          tunnel: [w2068 w2118] -> w2047
          tunnel: [w2067 w2117] -> w2046
          tunnel: w2045 -> [w2066 w2115]
          tunnel: [w2066 w2114] -> w2044
          tunnel: w2043 -> [w2065 w2113]
          tunnel: w2042 -> [w2064 w2112]
          tunnel: [w2065 w2111] -> w2041
          tunnel: [w2064 w2110] -> w2040
          tunnel: w2039 -> [w2063 w2109]
          tunnel: w2038 -> [w2062 w2108]
          tunnel: w2037 -> [w2061 w2107]
          tunnel: w2036 -> [w2060 w2106]
          tunnel: w2035 -> [w2059 w2105]
          tunnel: w2034 -> [w2058 w2104]
          tunnel: [w2063 w2103] -> w2033
          tunnel: [w2062 w2102] -> w2032
          tunnel: [w2061 w2101] -> w2031
          tunnel: [w2060 w2100] -> w2030
          tunnel: [w2059 w2099] -> w2029
          tunnel: [w2058 w2098] -> w2028
          tunnel: w2027 -> [w2076 w2097]
          tunnel: [w2076 w2096] -> w2026
          tunnel: [w2073 w2095] -> w2025
          tunnel: [w2072 w2094] -> w2024
          tunnel: [w2075 w2093] -> w2023
          tunnel: [w2071 w2092] -> w2022
          tunnel: [w2074 w2091] -> w2021
          tunnel: w2020 -> [w2075 w2090]
          tunnel: w2019 -> [w2074 w2089]
          tunnel: w2018 -> [w2073 w2088]
          tunnel: w2017 -> [w2072 w2087]
          tunnel: w2016 -> [w2071 w2086]
          tunnel: w2015 -> [_ w2085]
          tunnel: w2013 -> [w2057 w2084]
          tunnel: w2012 -> [w2056 w2083]
          tunnel: w2011 -> [w2055 w2082]
          tunnel: [w2057 w2081] -> w2010
          tunnel: [w2056 w2080] -> w2009
          tunnel: [w2055 w2079] -> w2008
          tunnel: w2007 -> [w2054 w2078]
          tunnel: [w2054 w2077] -> w2006
          frame False {
          }
          frame True {
            n1818 = Tick Count (ms)() -> (millisecond timer value=w2116:u32)
            n1819 = String To Byte Array(string=w2085) -> (unsigned byte array=w2129:u8[])
            n1820 = Array Size(array=w2129) -> (size(s)=w2128:i32)
            n1821 = formula code="// --- INTERNAL VARIABLE DECLARATIONS ---\nint i = 0;\nint phase = 0;\nint is_ch0_neg = 0;\nint is_ch1_neg = 0;\nint has_digits_0 = 0;\nint has_digits_1 = 0;\n\nint ch0_val = 0;    \nint ch1_val = 0;    \nfloat ch0_raw = 0.0;\nfloat ch1_raw = 0.0;\nfloat temp0 = 0.0;\nfloat temp1 = 0.0;\nfloat ch0_clean = 0.0;\nfloat ch1_clean = 0.0;\n\n// Temporary variables for P2P safety checks\nfloat calc_lvdt_min = 0.0;\nfloat calc_lvdt_max = 0.0;\nfloat calc_lvdt_p2p = 0.0;\nfloat calc_piezo_p2p = 0.0;\n\n// Median filter temporary variables\nfloat s0_0 = 0.0; float s0_1 = 0.0; float s0_2 = 0.0;\nfloat s1_0 = 0.0; float s1_1 = 0.0; float s1_2 = 0.0;\n\nfloat max_allowed_bits = 8388607.0;\n\n// --- STEP 1: DEFAULT TO HOLDING PREVIOUS VALUES ---\nout_LVDT_Min_V = in_LVDT_Min_V;\nout_LVDT_Max_V = in_LVDT_Max_V;\nout_LVDT_P2P_V = in_LVDT_P2P_V;\nout_Piezo_P2P  = in_Piezo_P2P;\nout_Friction_N = in_Friction_N;\nout_COF        = in_COF;\nwindow_ready   = 0;\n\n// --- STEP 2: PARSE INCOMING BYTE ARRAY ---\nif (array_size > 0) {\n    ch0_val = 0;\n    ch1_val = 0;\n    phase = 0;\n    is_ch0_neg = 0;\n    is_ch1_neg = 0;\n    has_digits_0 = 0;\n    has_digits_1 = 0;\n\n    for (i = 0; i < array_size; i++) {\n        if (raw_bytes[i] == 10 || raw_bytes[i] == 13) {\n            continue;\n        }\n\n        if (raw_bytes[i] == 45) { \n            if (phase == 0 && has_digits_0 == 0) {\n                is_ch0_neg = 1;\n            } else if (phase == 1 && has_digits_1 == 0) {\n                is_ch1_neg = 1;\n            }\n        } \n        else if (raw_bytes[i] == 59) { \n            phase = 1;\n        } \n        else if (raw_bytes[i] >= 48 && raw_bytes[i] <= 57) { \n            if (phase == 0) {\n                has_digits_0 = 1;\n                ch0_val = (ch0_val * 10) + (raw_bytes[i] - 48);\n            } else {\n                has_digits_1 = 1;\n                ch1_val = (ch1_val * 10) + (raw_bytes[i] - 48);\n            }\n        }\n    }\n\n    if (phase == 1 && has_digits_0 == 1 && has_digits_1 == 1) {\n        \n        ch0_raw = ch0_val * 1.0;\n        if (is_ch0_neg == 1) ch0_raw = ch0_raw * -1.0;\n\n        ch1_raw = ch1_val * 1.0;\n        if (is_ch1_neg == 1) ch1_raw = ch1_raw * -1.0;\n\n        if (ch0_raw > max_allowed_bits)  ch0_raw = max_allowed_bits;\n        if (ch0_raw < -max_allowed_bits) ch0_raw = -max_allowed_bits;\n        if (ch1_raw > max_allowed_bits)  ch1_raw = max_allowed_bits;\n        if (ch1_raw < -max_allowed_bits) ch1_raw = -max_allowed_bits;\n\n        // --- 3-SAMPLE MEDIAN FILTER ---\n        m0_2 = m0_1; m0_1 = m0_0; m0_0 = ch0_raw;\n        s0_0 = m0_0; s0_1 = m0_1; s0_2 = m0_2;\n        if (s0_0 > s0_1) { temp0 = s0_0; s0_0 = s0_1; s0_1 = temp0; }\n        if (s0_1 > s0_2) { temp0 = s0_1; s0_1 = s0_2; s0_2 = temp0; }\n        if (s0_0 > s0_1) { temp0 = s0_0; s0_0 = s0_1; s0_1 = temp0; }\n        ch0_clean = s0_1;\n\n        m1_2 = m1_1; m1_1 = m1_0; m1_0 = ch1_raw;\n        s1_0 = m1_0; s1_1 = m1_1; s1_2 = m1_2;\n        if (s1_0 > s1_1) { temp1 = s1_0; s1_0 = s1_1; s1_1 = temp1; }\n        if (s1_1 > s1_2) { temp1 = s1_0; s1_1 = s1_2; s1_2 = temp1; }\n        if (s1_0 > s1_1) { temp1 = s1_0; s1_0 = s1_1; s1_1 = temp1; }\n        ch1_clean = s1_1;\n\n        // --- CONTINUOUS MIN/MAX TRACKING ---\n        if (valid_samples == 0) {\n            min_ch0 = ch0_clean;\n            max_ch0 = ch0_clean;\n            min_ch1 = ch1_clean;\n            max_ch1 = ch1_clean;\n        } else {\n            if (ch0_clean > max_ch0) max_ch0 = ch0_clean;\n            if (ch0_clean < min_ch0) min_ch0 = ch0_clean;\n            if (ch1_clean > max_ch1) max_ch1 = ch1_clean;\n            if (ch1_clean < min_ch1) min_ch1 = ch1_clean;\n        }\n\n        valid_samples = valid_samples + 1;\n    }\n}\n\n// --- STEP 3: PEAK-HOLD WINDOW EVALUATION ---\nif (((current_time_ms - start_time_ms) >= 300) && (valid_samples >= 10)) {\n    \n    calc_lvdt_min = (min_ch0 * VREF) / 8388607.0;\n    calc_lvdt_max = (max_ch0 * VREF) / 8388607.0;\n    calc_lvdt_p2p = calc_lvdt_max - calc_lvdt_min;\n\n    calc_piezo_p2p = ((max_ch1 - min_ch1) * VREF) / 8388607.0;\n\n    // Update outputs continuously every 300ms window\n    out_LVDT_Min_V = calc_lvdt_min;\n    out_LVDT_Max_V = calc_lvdt_max;\n    out_LVDT_P2P_V = calc_lvdt_p2p;\n    \n    out_Piezo_P2P  = calc_piezo_p2p;\n    out_Friction_N = calc_piezo_p2p * PIEZO_CAL_FACTOR;\n    out_COF        = out_Friction_N / NORMAL_FORCE;\n    \n    window_ready   = 1;\n\n    // --- EXPONENTIAL DECAY (Fixes step-change latency) ---\n    // Slowly decay min/max outward by 10% towards ch0_clean instead of hard wiping.\n    // This allows real-time tracking when stroke amplitude expands (0.1 -> 0.2mm)\n    max_ch0 = max_ch0 - (max_ch0 - ch0_clean) * 0.10;\n    min_ch0 = min_ch0 + (ch0_clean - min_ch0) * 0.10;\n\n    max_ch1 = max_ch1 - (max_ch1 - ch1_clean) * 0.10;\n    min_ch1 = min_ch1 + (ch1_clean - min_ch1) * 0.10;\n\n    start_time_ms = current_time_ms;\n}"("raw_bytes"=w2129, "array_size"=w2128, "VREF"="VREF", "PIEZO_CAL_FACTOR"="PIEZO_CAL_FACTOR", "NORMAL_FORCE"="NORMAL_FORCE", "min_ch0"=w2124, "max_ch0"=w2123, "min_ch1"=w2122, "max_ch1"=w2121, "current_time_ms"=w2116, "start_time_ms"=w2115, "ch0_filt"=w2113, "ch1_filt"=w2112, "m0_0"=w2109, "m0_1"=w2108, "m0_2"=w2107, "m1_0"=w2106, "m1_1"=w2105, "m1_2"=w2104, "in_LVDT_Min_V"=w2097, "in_LVDT_Max_V"=w2090, "in_LVDT_P2P_V"=w2089, "in_Piezo_P2P"=w2088, "in_Friction_N"=w2087, "in_COF"=w2086, "hist_LVDT_P2P"=w2084, "hist_Friction"=w2083, "hist_COF"=w2082, "valid_samples"=w2078) -> ("window_ready"=→"Valid_data":dbl, "out_LVDT_Min_V"=w2096:dbl, "out_LVDT_Max_V"=w2095:dbl, "out_LVDT_P2P_V"=w2094:dbl, "out_Piezo_P2P"=w2093:dbl, "out_Friction_N"=w2092:dbl, "out_COF"=w2091:dbl, "min_ch0"=w2120:dbl, "max_ch0"=w2119:dbl, "min_ch1"=w2118:dbl, "max_ch1"=w2117:dbl, "start_time_ms"=w2114:u32, "ch0_filt"=w2111:dbl, "ch1_filt"=w2110:dbl, "m0_0"=w2103:dbl, "m0_1"=w2102:dbl, "m0_2"=w2101:dbl, "m1_0"=w2100:dbl, "m1_1"=w2099:dbl, "m1_2"=w2098:dbl, "hist_LVDT_P2P"=w2081:dbl, "hist_Friction"=w2080:dbl, "hist_COF"=w2079:dbl, "valid_samples"=w2077:dbl)
            "LVDT MIN" <- w2096
            "LVDT MAX" <- w2095
            "LVDT Peak" <- w2094
            "pizo raw" <- w2093
            "cof" <- w2091
            "Frictioin Force Raw" <- w2092
          }
        }
      }
      frame Error {
      }
    }
    n1822 = local read "Quit"() -> (w2005:bool)
  }
  n1823 = disable-structure shown="Enabled" {
    disable-tunnel: errorcluster {"status"=TRUE, "code"=0, "source"="Init"} ("error IO") -> [w2155 _]
    disable-tunnel: _ -> [w2154 _]
    frame Disabled {
    }
    frame Enabled {
    }
  }
  n1824 = while {
    stop <- w2165 stop-if-true
    # "V0OLTAGE TO STROKE (peice vise calibration)"
    n1825 = local read "LVDT MIN"() -> (w2157:dbl)
    n1826 = local read "LVDT Peak"() -> (w2156:dbl)
    n1827 = Wait (ms)(milliseconds to wait=u32 10) -> ()  [unwired: 1 out]
    n1828 = formula code="// Dynamic Parameterized Linear Interpolation Node\n// Inputs: vpp_val, voltages (Array), distances (Array)\n// Outputs: stroke\n\nint i = 0;\nint segments = 11; // 12 points make 11 interpolation segments\n\n// 1. Lower Boundary Clamp\nif (vpp_val <= voltages[0]) {\n    stroke = distances[0];\n}\n// 2. Upper Boundary Clamp\nelse if (vpp_val >= voltages[segments]) {\n    stroke = distances[segments];\n}\n// 3. Dynamic Segment Search Loop\nelse {\n    stroke = distances[0]; // Fallback baseline\n    for (i = 0; i < segments; i++) {\n        if (vpp_val >= voltages[i] && vpp_val <= voltages[i+1]) {\n            // Standard linear interpolation formula using array lookups\n            stroke = distances[i] + (vpp_val - voltages[i]) * (distances[i+1] - distances[i]) / (voltages[i+1] - voltages[i]);\n            break; // Segment found, safely exit the loop\n        }\n    }\n}"("vpp_val"=w2156, "voltages"="calibration values", "distances"="STROKE") -> ("stroke"=→"LVDT STROKE":dbl)
    n1829 = local read "Calibration Tare Value"() -> (w2161:dbl)
    n1830 = local read "Calibration Tare"() -> (w2159:bool)
    n1831 = Subtract(x=w2157, y=w2161) -> (x-y=→"LVDT STROKE  Calibration":dbl)
    n1832 = case shown="True" w2159 {
      selector: w2159 -> [_ w2167]
      tunnel: w2157 -> [_ w2168]
      frame False {
      }
      frame True {
        n1833 = Not(x=w2167) -> (.not. x?=w2166:bool)
        n1834 = local write "Calibration Tare"(w2166) -> ()
        "Calibration Tare Value" <- w2168
      }
    }
    n1835 = local read "Quit"() -> (w2165:bool)
  }
  n1836 = while {
    stop <- w2191 stop-if-true
    n1837 = local read "Due read"() -> (w2189:string)
    n1838 = call <vilib>:"High Resolution Polling Wait.vi"("seconds to wait"=0.02) -> ()  [unwired: 10 in, 1 out]
    n1839 = local read "Frictioin Force Raw"() -> (w2171:dbl)
    n1840 = Spreadsheet String To Array(delimiter (Tab)=";", format string="", spreadsheet string=w2189, array type (2D Dbl)=string[] []) -> (array=w2186:string[])
    n1841 = Fract/Exp String To Number(string=w2186) -> (number=w2185:dbl[])  [unwired: 3 in, 1 out]
    n1842 = call <vilib>:"Median Filter PtByPt.vi"("rank"=2, "x"=w2171) -> ("Filtered x"=→"Friction":dbl)  [unwired: 2 in, 1 out]
    n1843 = Index Array(array=w2185) -> (element #1=→"Sample Temperature 2":dbl, element #2=→"Target Sample Temperature":dbl, element #3=→"Current Duty Cycle":dbl, element #4=→"Ambient Temperature":dbl, element #5=→"Dac Status":dbl, element #6=→"Vpp":dbl, element #7=→"Active Error Code":dbl, element #8=→"Kp":dbl, element #9=→"Ki":dbl, element #10=→"Kd":dbl, element #11=→"SampleRaw":dbl, element #12=→"AmbRaw":dbl)  [unwired: 12 in]
    n1844 = local read "Quit"() -> (w2191:bool)
  }
  n1845 = while {
    shift-right: [w2205] -> w46
    shift-left: _ -> [w2197]
    shift-right: [w2192] -> w45
    shift-left: errorcluster {"status"=FALSE, "code"=0, "source"="Init"} ("error out") -> [w2199]
    tunnel: [w2194] -> w49
    tunnel: [w2204] -> _
    i -> [w2204]
    stop <- w2194 stop-if-true
    n1846 = local read "Com Port 2"() -> (w2198:refnum<visa-resource-name>)
    n1847 = local read "Port 2a"() -> (w2200:bool)
    n1848 = Unbundle(w2199) -> ("status"=→"Port 4":bool)  [unwired: 2 out]
    n1849 = call <vilib>:"High Resolution Polling Wait.vi"("seconds to wait"=0.02) -> ()  [unwired: 10 in, 1 out]
    n1850 = local read "Port 4"() -> (w2201:bool)
    n1851 = Not Equal?(x=w2198, y=w2197) -> (x != y?=w2196:bool)
    n1852 = Or(x=w2201, y=w2200) -> (x .or. y?=w2203:bool)
    n1853 = case shown="False" w2203 {
      frame False {
        w2208 = TRUE ("Visible")
        n1854 = property on="Port 2a" class="Bool (strict)"("Visible"=w2208) -> ()  [unwired: 2 in, 2 out]
        n1855 = property on="Port 4" class="Bool (strict)"("Visible"=w2208) -> ()  [unwired: 2 in, 2 out]
      }
      frame True {
        w2209 = TRUE ("Visible")
        n1856 = property on="Port 2a" class="Bool (strict)"("Visible"=w2209) -> ()  [unwired: 2 in, 2 out]
        n1857 = property on="Port 4" class="Bool (strict)"("Visible"=w2209) -> ()  [unwired: 2 in, 2 out]
      }
    }
    n1858 = case shown="True" w2196 {
      tunnel: [w2206 errorcluster {"status"=TRUE, "code"=0, "source"="Init"} ("error out")] -> w2195
      tunnel: w2199 -> [w2206 _]
      frame False {
      }
      frame True {
      }
    }
    n1859 = case shown="No Error" w2195 {
      selector: w2195 -> [w2222 w2253]
      tunnel: [w2215 w2258] -> w2205
      tunnel: [w2223 w2251] -> w2192
      tunnel: w2197 -> [w2224 w2256]
      frame No Error {
        n1860 = property class="Instr" props=["Serial Settings:Number of Bytes at Serial Port"](reference=w2224, error in=w2222) -> (reference out=w2216:refnum<visa-resource-name>, error out=w2221:errorcluster)  [unwired: 1 out]
        n1861 = while {
          tunnel: [w2232] -> w2217
          tunnel: [w2231] -> w2218
          tunnel: w2221 -> [w2230]
          tunnel: w2216 -> [w2229]
          tunnel: [w2228] -> _
          i -> [w2228]
          stop <- TRUE stop-if-true
          n1862 = property class="Instr" props=["Serial Settings:Number of Bytes at Serial Port"](reference=w2229, error in=w2230) -> (reference out=w2234:refnum<visa-resource-name>, error out=w2233:errorcluster)  [unwired: 1 out]
          n1863 = VISA Read(VISA resource name=w2234, byte count=u32 1000, error in (no error)=w2233) -> (VISA resource name out=w2231:refnum<visa-resource-name>, read buffer=→"Due read":string, error out=w2232:errorcluster)  [unwired: 1 out]
        }
        n1864 = local read "Due Write"() -> (w2214:string)
        n1865 = call <vilib>:"Trim Whitespace.vi"("string"=w2214) -> ("trimmed string"=w2213:string)  [unwired: 1 in]
        n1866 = Not Equal?(x=w2213, y="") -> (x != y?=w2219:bool)
        n1867 = VISA Flush I/O Buffer(VISA resource name=w2218) -> (VISA resource name out=w2211:refnum<visa-resource-name>, error out=→"error out 10":errorcluster)  [unwired: 2 in]
        n1868 = case shown="True" w2219 {
          tunnel: w2211 -> [w2236 w2241]
          tunnel: [w2236 w2245] -> w2215
          tunnel: w2217 -> [w2235 w2240]
          tunnel: [w2235 w2243] -> w2223
          tunnel: w2213 -> [_ w2239]
          tunnel: [_ w2242] -> _
          frame False {
            # "DATA  WRITE LOOP"
          }
          frame True {
            n1869 = Concatenate Strings(w2239, "\r\n") -> (w2238:string)
            n1870 = VISA Write(VISA resource name=w2241, write buffer=w2238, error in (no error)=w2240) -> (VISA resource name out=w2245:refnum<visa-resource-name>, return count=w2242:u32, error out=w2244:errorcluster)
            n1871 = flat-sequence {
              tunnel: w2244 -> [w2247]
              tunnel: [w2247] -> w2243
              frame #0 {
                n1872 = local write "Due Write"("" ("Command")) -> ()
                n1873 = Wait (ms)(milliseconds to wait=u32 5) -> ()  [unwired: 1 out]
              }
            }
          }
        }
        "Port 2a" <- TRUE ("Port 2a")
      }
      frame Error {
        w2264 = u16 0 items=["None", "XON/XOFF", "RTS/CTS", "XON/XOFF & RTS/CTS", "DTR/DSR", "XON/XOFF & DTR/DSR"] ("flow control (0:none)  2")
        w2262 = u16 10 items=["1.0"=10, "1.5"=15, "2.0"=20] ("stop bits 2")
        w2260 = u16 0 items=["None", "Odd", "Even", "Mark", "Space"] ("parity 2")
        w2261 = u32 10000  # timeout (10sec)
        n1874 = VISA Clear(VISA resource name=w2256, error in (no error)=w2253) -> (VISA resource name out=w2255:refnum<visa-resource-name>, error out=w2254:errorcluster)
        n1875 = VISA Close(VISA resource name=w2255, error in (no error)=w2254) -> (error out=w2257:errorcluster)
        n1876 = call <vilib>:"Clear Errors.vi"("error in (no error)"=w2257) -> ()  [unwired: 5 in, 2 out]
        n1877 = local write "Port 2a"(FALSE ("Port 2a")) -> ()
        n1878 = local read "Com Port 2"() -> (w2250:refnum<visa-resource-name>)
        "visa due" <- w2250
        n1879 = call-poly "VISA Configure Serial Port"("VISA resource name"=w2250, "timeout (10sec)"=w2261, "baud rate (9600)"=u32 250000 ("baud rate  2"), "data bits (8)"=u16 8 ("data bits  2"), "parity (0:none)"=w2260, "stop bits (10: 1 bit)"=w2262, "flow control (0:none)"=w2264) -> ("VISA resource name out"=w2265:refnum<visa-resource-name>, "error out"=w2266:errorcluster)  [unwired: 7 in]
        n1880 = flat-sequence {
          tunnel: w2265 -> [w2268]
          tunnel: w2266 -> [w2267]
          tunnel: [w2268] -> w2258
          tunnel: [w2267] -> w2251
          frame #0 {
            n1881 = Wait (ms)(milliseconds to wait=u32 50) -> ()  [unwired: 1 out]
          }
        }
        "Residual Due" <- ""
      }
    }
    "error out 9" <- w2192
    n1882 = local read "Quit"() -> (w2194:bool)
    "Error Due" <- w2199
  }
  n1883 = local write "FRICVALZ"(0.0 ("FRICVALZ")) -> ()
  n1884 = property on="RUN" class="Bool (strict)"("Visible"=TRUE) -> ()  [unwired: 2 in, 2 out]
  n1885 = while {
    tunnel: [w2283] -> _
    tunnel: [w2270] -> w57
    i -> [w2283]
    stop <- w2270 stop-if-true
    n1886 = local read "conststatus"() -> (w2274:dbl)
    n1887 = local read "Main Tab"() -> (w2272:T4)
    n1888 = local read "EDIT"() -> (w2289:bool)
    n1889 = local read "Rate"() -> (w2288:dbl)
    n1890 = case shown="True" w2289 {
      tunnel: [FALSE TRUE] -> _
      frame False {
      }
      frame True {
      }
    }
    n1891 = Equal?(x=w2272, y=T29."About" ("Main Tab")) -> (x = y?=w2281:bool)
    n1892 = Equal?(x=w2274, y=0.0) -> (x = y?=w2275:bool)
    n1893 = Divide(x=1.0, y=w2288) -> (x/y=w2284:dbl)
    "Time 2" <- w2284
    n1894 = case shown="True" w2275 {
      frame False {
      }
      frame True {
        # "C:\\WinDucom\\calibrate WO 2391.dcf"
        n1895 = local write "Lan flag"(22) -> ()
        n1896 = local write "conststatus"(10.0 ("rpm value : 2")) -> ()
        n1897 = String To Path(string="C:\\LAB-IQ\\calibrate WO 2472.dcf") -> (path=w2295:path)
        n1898 = Open/Create/Replace File "Open File"(file path (use dialog)=w2295) -> (refnum out=w2293:refnum<file>)  [unwired: 5 in, 2 out]
        n1899 = for {
          N: 23 -> [_]
          tunnel: w2293 -> [w2304]
          i -> [w2298]
          (unwired) TRUE ("line mode (F)")
          n1900 = Read from Text File "Read File"(file (use dialog)=w2304) -> (text=w2303:string)  [unwired: 3 in, 3 out]
          n1901 = Match Pattern(string=w2303, regular expression="]") -> (after substring=w2301:string)  [unwired: 1 in, 3 out]
          n1902 = String Subset(string=w2303, offset (0)=5, length (rest)=10 ("length (rest)")) -> (substring=w2296:string)
          n1903 = Fract/Exp String To Number(string=w2296) -> (number=w2297:dbl)  [unwired: 3 in, 1 out]
          n1904 = Match Pattern(string=w2301, regular expression="-") -> (before substring=w2299:string)  [unwired: 1 in, 3 out]
          n1905 = case shown="10" w2298 {
            tunnel: w2297 -> [_ _ _ _ _ _ _ _ _ _ w2311 _ _ _ _ _ _ _ _ _ _ _ _ _]
            tunnel: w2299 -> [_ _ _ _ w2307 w2308 w2309 _ _ _ _ _ _ _ _ _ _ _ _ _ w2312 w2313 w2314 _]
            frame 0 {
            }
            frame 1 {
            }
            frame 2 {
            }
            frame 3 {
            }
            frame 4 {
              n1906 = local write "Com Port 1"(w2307) -> ()
            }
            frame 5 {
              n1907 = local write "Com Port 2"(w2308) -> ()
              n1908 = local write "visa due"(w2308) -> ()
            }
            frame 6 {
              n1909 = String To Path(string=w2309) -> (path=w2310:path)
              n1910 = local write "File Path"(w2310) -> ()
              "String" <- w2309
            }
            frame 7 {
            }
            frame 8 {
            }
